vi "Measurement Template(Old).vi"(8 "error in (no error)":errorcluster, 11 "measurement configuration":cluster{}) -> (0 "error out":errorcluster, 3 "measurement results":cluster{})   [LabVIEW 2021]
uses:
  <vilib>/gRPC/LabVIEW gRPC Library/grpc-lvsupport-release.lvlib
  Runtime/Clients/Measurement Service Client V2/Measurement Service Client V2.lvlib
  35f71eb9-7158-4110-bfb1-6d749e6fa8f4.vi
  Runtime/Clients/Measurement Client V2/Client.lvlib
  ef0035e8-05ef-469b-9be2-5e457b1f40d8.vi
  Runtime/Clients/Measurement Service Client V2/RPC Messages/ni_measurementlink_measurement_v2_MeasureRequest.ctl
  Runtime/Clients/Measurement Service Client V2/RPC Messages/ni_measurementlink_PinMapContext.ctl
  Runtime/Clients/Measurement Service Client V2/RPC Messages/google_protobuf_Any.ctl
panel:
  in  "stop":bool
  in  "service class":string="Voltage Measurement_LabVIEW"
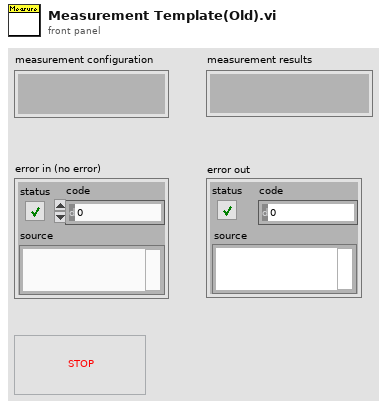
[diagram p1: front panel]
types:
  T1 = typedef "Measurement Service Client V2.lvlib/ni_measurementlink_measurement_v2_MeasureRequest.ctl" = cluster{"configuration_parameters":T2, "pin_map_context":T3}
  T2 = typedef "Measurement Service Client V2.lvlib/google_protobuf_Any.ctl" = cluster{"type_url":string, "value":u8[]}
  T3 = typedef "Measurement Service Client V2.lvlib/ni_measurementlink_PinMapContext.ctl" = cluster{"pin_map_id":string, "sites":i32[]}
  T4 = typedef "grpc-lvsupport-release.lvlib/grpcId.ctl" = u64
  T5 = typedef "grpc-lvsupport-release.lvlib/Message Metadata.ctl" = cluster{"Version":i32, "Name":string, "Type Url":string, "Elements":T6[], "Has Oneof":bool}
  T6 = typedef "grpc-lvsupport-release.lvlib/Message Element Metadata.ctl" = cluster{"Field Name":string, "Embedded Message Name":string, "Protobuf Index":i32, "MessageElementType":T7, "Repeated":bool, "Is in Oneof":bool, "Oneof Container Name":string}
  T7 = typedef "grpc-lvsupport-release.lvlib/Message Element Type.ctl" = enum32{"Int32Value", "FloatValue", "DoubleValue", "BoolValue", "StringValue", "MessageValue", "Int64Value", "UInt32Value", "UInt64Value", "EnumValue", "Bytes", "Fixed64", "Fixed32", "SFixed64", "SFixed32", "SInt64", "SInt32"}
  T8 = typedef "grpc-lvsupport-release.lvlib/Any.ctl" = cluster{"Type Url":string, "Bytes":u8[]}
  T9 = typedef "Measurement Service Client V2.lvlib/ni_measurementlink_measurement_v2_MeasureResponse.ctl" = cluster{"outputs":T2}
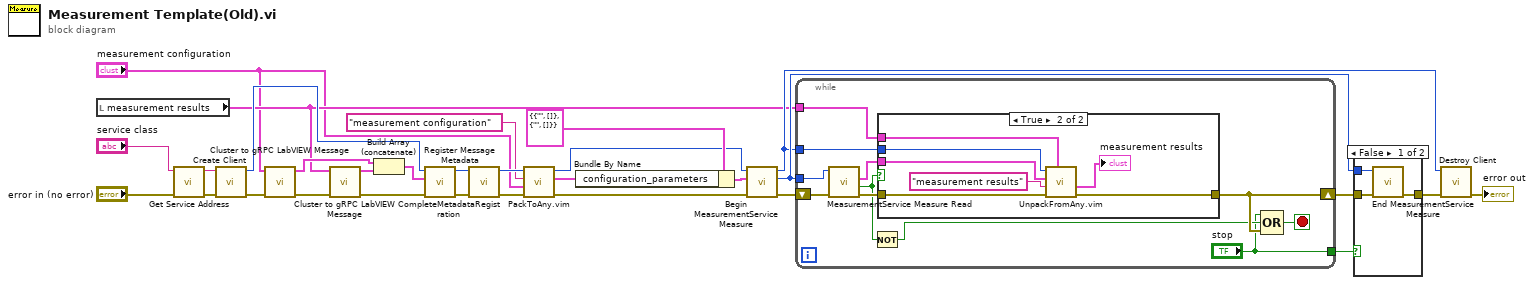
[diagram p0: block diagram]
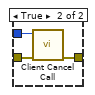
[diagram p2: hidden frame]
diagram:
  n1 = local read "measurement results"() -> (w3:cluster{})
  n2 = call "Get Service Address.vi"("error in"="error in (no error)", "service to run"="service class") -> ("error out"=w19:errorcluster, "service address"=w17:string)  [unwired: 8 in]
  n3 = call "Create Client.vi"("error in"=w19, "address"=w17) -> ("error out"=w16:errorcluster, "gRPC ID Out"=w15:T4)  [unwired: 8 in]
  n4 = call <vilib>:"Cluster to gRPC LabVIEW Message.vi"("error in"=w16, "Cluster"="measurement configuration") -> ("error out"=w21:errorcluster, "gRPC Message Metadata []"=w30:T5[])  [unwired: 7 in, 1 out]
  n5 = call <vilib>:"Cluster to gRPC LabVIEW Message.vi"("error in"=w21, "Cluster"=w3) -> ("error out"=w20:errorcluster, "gRPC Message Metadata []"=w29:T5[])  [unwired: 7 in, 1 out]
  n6 = Build Array (concatenate)(w30, w29) -> (w28:T5[])
  n7 = call <vilib>:"Register Message Metadata.vi"("error in"=w20, "Messages"=w28, "gRPCid in"=w15) -> ("error out"=w27:errorcluster, "gRPCid out"=w14:T4)  [unwired: 7 in]
  n8 = call <vilib>:"CompleteMetadataRegistration.vi"("error in"=w27, "gRPC ID in"=w14) -> ("error out"=w22:errorcluster, "gRPC ID Out"=w13:T4)  [unwired: 8 in]
  n9 = call "PackToAny.vim"("error in"=w22, "Data To Pack"="measurement configuration", "Message Type"="measurement configuration", "gRPCid in"=w13) -> ("error out"=w26:errorcluster, "Any"=w24:T8, "gRPCid out"=w5:u64)  [unwired: 5 in]
  n10 = Bundle By Name(cluster=T1 {"configuration_parameters"={"type_url"="", "value"=[]}, "pin_map_context"={"pin_map_id"="", "sites"=[]}} ("Request Data"), "configuration_parameters"=w24) -> (w23:T1)
  n11 = call "Begin MeasurementService Measure.vi"("error in"=w26, "Request Data"=w23, "gRPC ID"=w5) -> ("error out"=w8:errorcluster, "Call Id Out"=w7:T4, "gRPC ID out"=w6:T4)  [unwired: 6 in]
  n12 = while {
    tunnel: w7 -> [w38]
    tunnel: w6 -> [w37]
    shift-right: [w35] -> w10
    shift-left: w8 -> [w39]
    tunnel: ["stop"] -> w11
    tunnel: w3 -> [w31]
    stop <- w41 stop-if-true
    n13 = call "MeasurementService Measure Read.vi"("error in"=w39, "Call ID in"=w38) -> ("error out"=w36:errorcluster, "Success"=w34:bool, "Response Data"=w40:T9)  [unwired: 6 in, 1 out]
    n14 = Not(x=w34) -> (.not. x?=w33:bool)
    n15 = case shown="True" w34 {
      tunnel: w40 -> [_ w49]
      tunnel: w37 -> [_ w48]
      tunnel: w36 -> [w42 w47]
      tunnel: [w42 w46] -> w35
      tunnel: w31 -> [_ w44]
      frame False {
      }
      frame True {
        n16 = call "UnpackFromAny.vim"("Data Type"=w44, "error in"=w47, "Message Type"="measurement results", "Any"=w49, "gRPCid in"=w48) -> ("error out"=w46:errorcluster, "Unpacked Value"=→"measurement results":cluster{"Measurement from SMU Str 2":string})  [unwired: 4 in, 1 out]
      }
    }
    n17 = Compound Arithmetic op=OR("stop", w33, w35) -> (w41:bool)
  }
  n18 = case shown="False" w11 {
    tunnel: w7 -> [w51 w55]
    tunnel: w10 -> [w52 w54]
    tunnel: [w50 w53] -> w9
    frame False {
      n19 = call "End MeasurementService Measure.vi"("error in"=w52, "Call ID in"=w51) -> ("error out"=w50:errorcluster)  [unwired: 8 in, 1 out]
    }
    frame True {
      n20 = call <vilib>:"Client Cancel Call.vi"("error in"=w54, "Call ID in"=w55) -> ("error out"=w53:errorcluster)  [unwired: 7 in, 2 out]
    }
  }
  n21 = call "Destroy Client.vi"("error in"=w9, "gRPC ID"=w6) -> ("error out"=→"error out":errorcluster)  [unwired: 9 in]
